vi "FT Controls Change.vi"(8 "error in (no error)":errorcluster, 9 "F/T Controls Cluster Variant":variant, 11 "Rigol DG822 Pulse in":refnum<class "Rigol DG822 Pulse.lvclass">) -> (0 "error out":errorcluster, 1 "New F/T Controls Cluster Variant":variant, 3 "Rigol DG822 Pulse out":refnum<class "Rigol DG822 Pulse.lvclass">)   [LabVIEW 2021, in "Rigol DG822 UI.lvlib" / "Rigol DG822 Pulse.lvlib" / "Rigol DG822 Pulse.lvclass"]
uses:
  Rigol DG822 Pulse.lvclass
  Rigol DG822 UI/lib/controls.llb/FT Controls Cluster.ctl
  Rigol DG822 Pulse.lvclass/Rigol DG822 Pulse.ctl
  General/Files/lvlibp/Actors.lvlibp/Actors/Actors/Actors.lvclass
  D:/LabVIEW/General/Files/lvlibp/Actors.lvlibp/Actors/Actors/Actors.lvclass
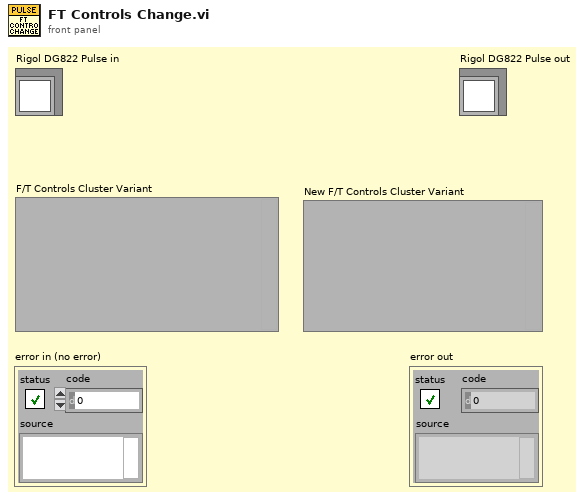
[diagram p1: front panel]
types:
  T1 = typedef "FT Controls Cluster.ctl" = cluster{"Freq/Period":bool, "Ampl/HighL":bool, "Offset/LowL":bool, "Duty/Width":bool}
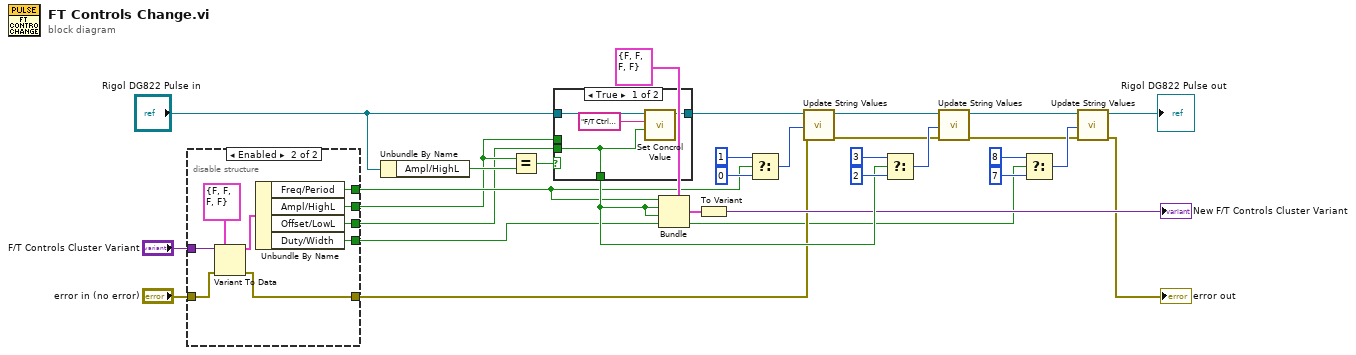
[diagram p0: block diagram]
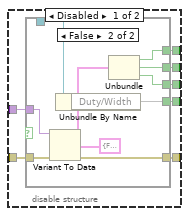
[diagram p2: hidden frame]
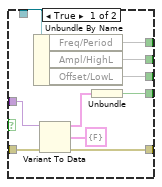
[diagram p3: hidden frame]
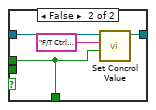
[diagram p4: hidden frame]
diagram:
  n1 = disable-structure shown="Enabled" {
    disable-tunnel: "F/T Controls Cluster Variant" -> [w37 w66]
    disable-tunnel: "error in (no error)" -> [w36 w65]
    disable-tunnel: [w35 w64] -> w13
    disable-tunnel: [w34 w61] -> w12
    disable-tunnel: [w33 w60] -> w11
    disable-tunnel: [w32 w58] -> w10
    disable-tunnel: [w31 w59] -> w2
    frame Disabled {
      n2 = case shown="False" {
        selector: _ -> [_ _]
        tunnel: w37 -> [w47 w57]
        tunnel: w36 -> [w46 w56]
        tunnel: _ -> [w45 w54]
        tunnel: [w44 w50] -> w34
        tunnel: [w43 w49] -> w33
        tunnel: [w42 w48] -> w32
        tunnel: [w38 w53] -> w31
        tunnel: [w41 w52] -> w35
        frame True {
          n3 = Unbundle By Name(w45) -> ("Freq/Period"=w44, "Ampl/HighL"=w43, "Offset/LowL"=w42)
          n4 = Variant To Data(error in=w46, type=cluster{bool} {FALSE}, Variant=w47) -> (data=w39:cluster{bool}, error out=w41:errorcluster)
          n5 = Unbundle(w39) -> (w38:bool)
        }
        frame False {
          n6 = Variant To Data(error in=w56, type=cluster{bool, bool, bool} {FALSE, FALSE, FALSE}, Variant=w57) -> (data=w51:cluster{bool, bool, bool}, error out=w52:errorcluster)
          n7 = Unbundle By Name(w54) -> ("Duty/Width"=w53)
          n8 = Unbundle(w51) -> (w50:bool, w49:bool, w48:bool)
        }
      }
    }
    frame Enabled {
      n9 = Variant To Data(error in=w65, type=T1 {"Freq/Period"=FALSE, "Ampl/HighL"=FALSE, "Offset/LowL"=FALSE, "Duty/Width"=FALSE} ("F/T Ctrls"), Variant=w66) -> (data=w62:T1, error out=w64:errorcluster)
      n10 = Unbundle By Name(w62) -> ("Freq/Period"=w61:bool, "Ampl/HighL"=w60:bool, "Offset/LowL"=w58:bool, "Duty/Width"=w59:bool)
    }
  }
  n11 = Unbundle By Name("Rigol DG822 Pulse in") -> ("Ampl/HighL"=w16:bool)
  n12 = Equal?(x=w11, y=w16) -> (x = y?=w19:bool)
  n13 = case shown="True" w19 {
    tunnel: [w70 w74] -> w24
    tunnel: "Rigol DG822 Pulse in" -> [w68 w72]
    tunnel: w10 -> [w67 _]
    tunnel: w11 -> [_ w71]
    tunnel: [w67 w71] -> w20
    frame True {
      n14 = call "Set Concrol Value.vi"("Value"=w67, "Control Label"="F/T Ctrls.Ampl/HighL", "Actors in"=w68) -> ("Actors out"=w70:refnum<class "Rigol DG822 Pulse.lvclass">)  [unwired: 7 in, 1 out]
    }
    frame False {
      n15 = call "Set Concrol Value.vi"("Value"=w71, "Control Label"="F/T Ctrls.Offset/LowL", "Actors in"=w72) -> ("Actors out"=w74:refnum<class "Rigol DG822 Pulse.lvclass">)  [unwired: 7 in, 1 out]
    }
  }
  n16 = Bundle(cluster=T1 {"Freq/Period"=FALSE, "Ampl/HighL"=FALSE, "Offset/LowL"=FALSE, "Duty/Width"=FALSE} ("F/T Ctrls"), "Freq/Period"=w12, "Ampl/HighL"=w20, "Offset/LowL"=w20, "Duty/Width"=w2) -> (w30:T1)
  n17 = To Variant(anything=w30) -> (Variant=→"New F/T Controls Cluster Variant":variant)
  n18 = Select(t=u16 1 ("Type"), s=w12, f=u16 0) -> (s? t:f=w27:u16)
  n19 = call-dynamic "Update String Values.vi"("error in (no error)"=w13, "Type"=w27, "Rigol DG822 Pulse in"=w24) -> ("error out"=w21:errorcluster, "Rigol DG822 Pulse out"=w22:refnum<class "Rigol DG822 Pulse.lvclass">)  [unwired: 7 in]
  n20 = Select(t=u16 3 ("Type"), s=w20, f=u16 2) -> (s? t:f=w23:u16)
  n21 = call-dynamic "Update String Values.vi"("error in (no error)"=w21, "Type"=w23, "Rigol DG822 Pulse in"=w22) -> ("error out"=w3:errorcluster, "Rigol DG822 Pulse out"=w4:refnum<class "Rigol DG822 Pulse.lvclass">)  [unwired: 7 in]
  n22 = Select(t=u16 8 ("Type"), s=w2, f=u16 7) -> (s? t:f=w8:u16)
  n23 = call-dynamic "Update String Values.vi"("error in (no error)"=w3, "Type"=w8, "Rigol DG822 Pulse in"=w4) -> ("error out"=→"error out":errorcluster, "Rigol DG822 Pulse out"=→"Rigol DG822 Pulse out":refnum<class "Rigol DG822 Pulse.lvclass">)  [unwired: 7 in]
